vi "ResonanceAnalyzer.vi"() -> ()   [LabVIEW 2015]
uses:
  <vilib>/imath/engines/lvmath2/RunTimeEngine/RangeToken/NIMS_Range_R2 - Float.vi
  <instcachedir>/0/NIMS_Range_R2 - Float_98052C3F8D284261A146188355820AF0.lvgen/NIMS_Range_R2 - Float_98052C3F8D284261A146188355820AF0_000.vi
  <vilib>/imath/engines/lvmath2/RunTimeEngine/CommandStatement/MC_CommandStatement_break.vi
  <vilib>/imath/engines/lvmath2/RunTimeEngine/RowToken/NIMS_RowToken_M_SorRV.vi
  <instcachedir>/0/NIMS_RowToken_M_SorRV_0ECFFCDE6465458AAAF8A8ED2D6C8AF1.lvgen/NIMS_RowToken_M_SorRV_0ECFFCDE6465458AAAF8A8ED2D6C8AF1_002.vi
  <vilib>/imathl/engines/lvmath/Functions/Error Handling/Create Error.vi
  <vilib>/imath/engines/lvmath2/RunTimeEngine/NodeEndStatement/NIMS_NodeEndStatement_Get Vector.vi
  <instcachedir>/0/NIMS_NodeEndStatement_Get Vector_ED7FC4F6B50246F79D573C75B2E51AF8.lvgen/NIMS_NodeEndStatement_Get Vector_ED7FC4F6B50246F79D573C75B2E51AF8_001.vi
  <vilib>/imath/engines/lvmath/Functions/Error Handling/MergeErrorsWrapper.vi
  <vilib>/imath/engines/lvmath2/RunTimeEngine/NodeEndStatement/NIMS_NodeEndStatement_Output.vi
  <instcachedir>/0/NIMS_NodeEndStatement_Output_53EC0D466D134D7ABD903AC30B43404B.lvgen/NIMS_NodeEndStatement_Output_53EC0D466D134D7ABD903AC30B43404B_005.vi
  <vilib>/imath/engines/lvmath2/RunTimeEngine/ErrorHandling/NIMS_Finalize Error.vi
  <vilib>/Utility/file.llb/Read Delimited Spreadsheet (DBL).vi
panel:
  out "XY Graph":cluster{"freq":dbl[], "L":dbl[]}(graph)
  in  "Tab Control":enum32{"Simulated", "Experiment"}(tab)
  in  "Q":dbl
  in  "Center Freq":dbl
  in  "Start Freq":dbl
  in  "End Freq":dbl
  in  "df":dbl
  in  "Noise Level":dbl
  in  "Filename":path
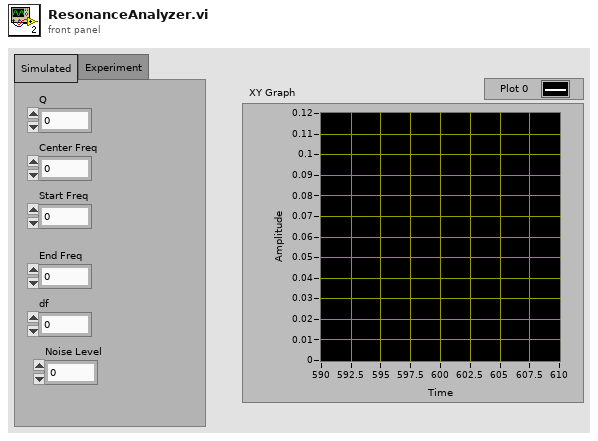
[diagram p1: front panel]
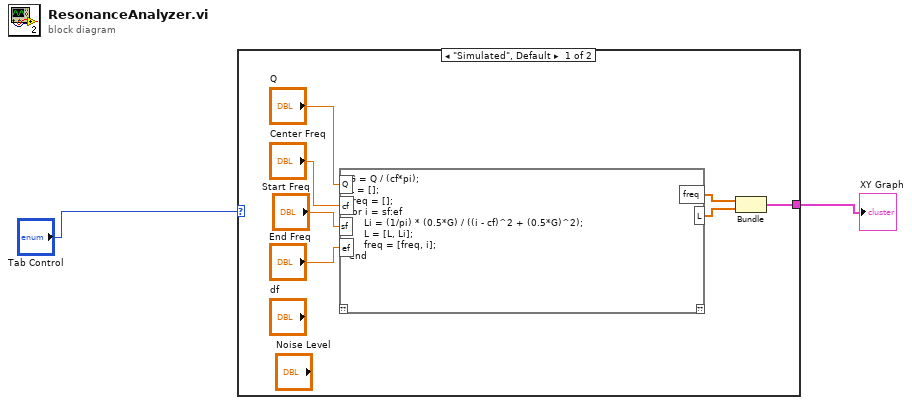
[diagram p0: block diagram]
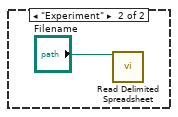
[diagram p2: hidden frame]
diagram:
  n1 = case shown="\"Simulated\", Default" "Tab Control" {
    tunnel: [w3 _] -> w1
    frame "Simulated", Default {
      n2 = mathscript code="G = Q / (cf*pi);\nL = [];\nfreq = [];\nfor i = sf:ef \n     Li = (1/pi) * (0.5*G) / ((i - cf)^2 + (0.5*G)^2);\n     L = [L, Li];\n     freq = [freq, i];\nend"("cf"="Center Freq", "Q"="Q", "sf"="Start Freq", "ef"="End Freq") -> ("freq"=w5:dbl[], "L"=w4:dbl[])  [unwired: 1 in, 1 out]
      n3 = Bundle("freq"=w5, "L"=w4) -> (w3:cluster{"freq":dbl[], "L":dbl[]})  [unwired: 1 in]
    }
    frame "Experiment" {
      n4 = call-poly <vilib>:"Read Delimited Spreadsheet.vi"("file path (dialog if empty)"="Filename") -> ()  [unwired: 9 in, 6 out]
    }
  }
  "XY Graph" <- w1
